vi "Get Single-Line Package Attribute Value.vi"(8 "error in (no error)":errorcluster, 10 "package attribute name":string, 11 "package attributes CLI string":string) -> (0 "error out":errorcluster, 1 "attribute found?":bool, 3 "package attribute value":string)   [LabVIEW 2014, in "NIPM_API.lvlib"]
uses:
  NIPM_API.lvlib
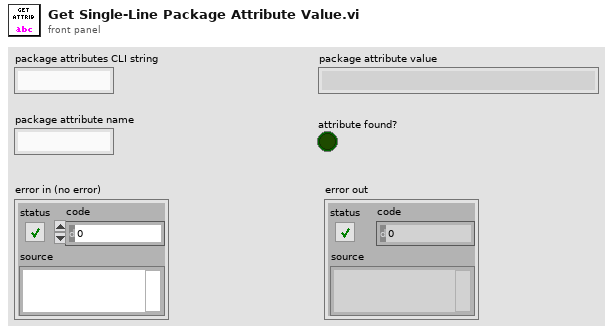
[diagram p1: front panel]
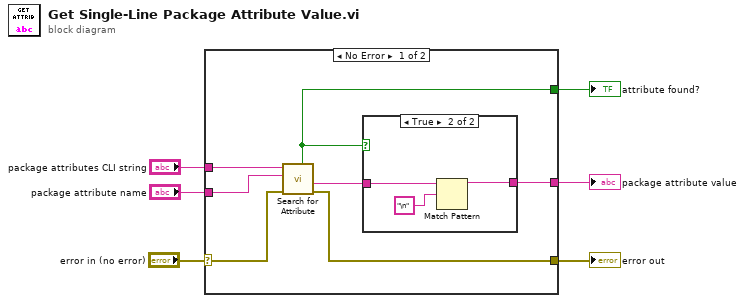
[diagram p0: block diagram]
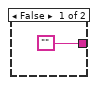
[diagram p2: hidden frame]
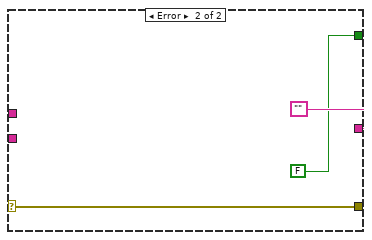
[diagram p3: hidden frame]
diagram:
  n1 = case shown="No Error" "error in (no error)" {
    selector: "error in (no error)" -> [w10 w20]
    tunnel: [w12 "" ("package attribute CLI string")] -> w6
    tunnel: "package attribute name" -> [w11 _]
    tunnel: "package attributes CLI string" -> [w13 _]
    tunnel: [w9 w20] -> w2
    tunnel: [w8 FALSE] -> w1
    frame No Error {
      n2 = call "Search for Attribute.vi"("error in (no error)"=w10, "package attribute name"=w11, "package attributes CLI string in"=w13) -> ("error out"=w9:errorcluster, "string after attribute"=w7:string, "attribute found?"=w8:bool)  [unwired: 3 in, 3 out]
      n3 = case shown="True" w8 {
        tunnel: w7 -> [_ w16]
        tunnel: ["" w15] -> w12
        frame False {
        }
        frame True {
          n4 = Match Pattern(string=w16, regular expression="\n") -> (before substring=w15:string)  [unwired: 1 in, 3 out]
        }
      }
    }
    frame Error {
    }
  }
  "package attribute value" <- w6
  "error out" <- w2
  "attribute found?" <- w1
